vi "Write Log record configuration.vi"(8 "error in (no error)":errorcluster, 10 "Configuration":T1={"OSF node  ID"="", "Conection timeout"=60.0, "Station"="", "Log server "="magx", "Upload to OSF"=FALSE, "Append to lab book"=FALSE} {"Conection timeout" format="%#_6ps"}, 11 "Log Record in":refnum<class "Log Record.lvclass">) -> (0 "error out":errorcluster, 3 "Log Record out":refnum<class "Log Record.lvclass">)   [LabVIEW 2020, in "Log Record.lvclass"]
uses:
  Log Record.lvclass
  C:/GitHub/LabActor/Template Module/Template Module.lvclass
  Log Record Configuration.ctl
  Template Module/Template Module.lvclass/Template Module.ctl
  Template Module/Write Configuration.vi
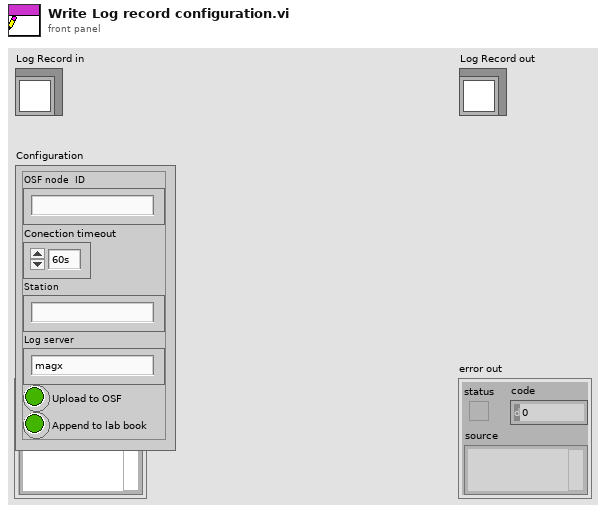
[diagram p1: front panel]
types:
  T1 = typedef "Log Record Configuration.ctl" = cluster{"OSF node  ID":string, "Conection timeout":dbl, "Station":string, "Log server ":string, "Upload to OSF":bool, "Append to lab book":bool}
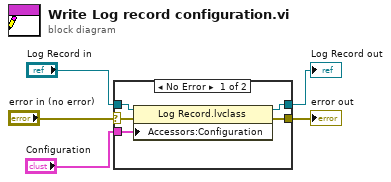
[diagram p0: block diagram]
diagram:
  n1 = case shown="No Error" "error in (no error)" {
    selector: "error in (no error)" -> [w10 w11]
    tunnel: [w9 w11] -> w4
    tunnel: [w7 w12] -> w2
    tunnel: "Log Record in" -> [w8 w12]
    tunnel: "Configuration" -> [w6 _]
    frame No Error {
      n2 = property class="Log Record.lvclass"(reference=w8, error in=w10, "Accessors:Configuration"=w6) -> (reference out=w7:refnum<class "Log Record.lvclass">, error out=w9:errorcluster)
    }
    frame Error {
    }
  }
  "error out" <- w4
  "Log Record out" <- w2
